vi "Periodic Tasks.vi"(8 "error in":errorcluster) -> ()   [LabVIEW 2013]
doc: "This VI runs in parallel to other tasks. It can contain as many user-defined periodic loops as you need. These can carry out PID or other sorts of timed response."
uses:
  <vilib>/Rock Robotics/WPI/DriverStation/WPI_DriverStationRobotMode2.ctl
  <vilib>/Rock Robotics/SystemInterfaces/Utilities/FPGA_UtilitiesLED Source.ctl
  <vilib>/Rock Robotics/SystemInterfaces/Utilities/FPGA_UtilitiesLED State.ctl
  <vilib>/Rock Robotics/WPI/Solenoid/WPI_SolenoidValue.ctl
  <vilib>/Rock Robotics/WPI/Relay/WPI_RelayValue.ctl
  <vilib>/Rock Robotics/WPI/Compressor/WPI_CompressorGetSetRefNum.vi
  Robot Global Data.vi
  <vilib>/Rock Robotics/WPI/Joystick/WPI_JoystickGetSetRefNum.vi
  <vilib>/Rock Robotics/WPI/Solenoid/WPI_SolenoidSetEnum.vi
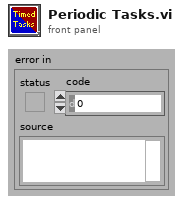
[diagram p1: front panel]
types:
  T1 = typedef "FPGA_UtilitiesLED State.ctl" = enum16{"Off", "On", "Toggle"}
  T2 = typedef "FPGA_UtilitiesLED Source.ctl" = enum16{"User LED", "FPGA LED"}
  T3 = typedef "WPI_AnalogChannelDevRef.ctl" = cluster{"DevStatus":errorcluster, "Analog Module":T4, "Analog Channel":T5}
  T4 = typedef "FPGA_TypedefAnalogModule.ctl" = enum16{"Analog Module 1", "Analog Module 2"}
  T5 = typedef "FPGA_AIChannel.ctl" = enum8{"AI 1", "AI 2", "AI 3", "AI 4", "AI 5", "AI 6", "AI 7", "AI 8", "Invalid"}
  T6 = typedef "WPI_RelayDevRef.ctl" = cluster{"DevStatus":errorcluster, "Relay Channel":T7, "Digital Module":T8, "Relay Direction":T9}
  T7 = typedef "FPGA_DIORelayChannel.ctl" = enum8{"Relay 1", "Relay 2", "Relay 3", "Relay 4", "Relay 5", "Relay 6", "Relay 7", "Relay 8", "Invalid"}
  T8 = typedef "FPGA_TypedefDigitalModule.ctl" = enum16{"Digital Module 1", "Digital Module 2"}
  T9 = typedef "WPI_RelayDirection.ctl" = enum16{"Both directions", "Forward only", "Reverse only"}
  T10 = typedef "WPI_DigitalInputDevRef.ctl" = cluster{"DevStatus":errorcluster, "DIO Channel":T11, "Digital Module":T8}
  T11 = typedef "FPGA_DIOChannel.ctl" = enum8{"DIO 1", "DIO 2", "DIO 3", "DIO 4", "DIO 5", "DIO 6", "DIO 7", "DIO 8", "DIO 9", "DIO 10", "DIO 11", "DIO 12", "DIO 13", "DIO 14", "Invalid"}
  T12 = typedef "WPI_SolenoidDevRef.ctl" = cluster{"DevStatus":errorcluster, "Solenoid Module":T13, "Forward Solenoid Channel":T14, "Reverse Solenoid Channel":T14}
  T13 = typedef "FPGA_TypedefSolenoidModule.ctl" = enum16{"Solenoid Module 1", "Solenoid Module 2"}
  T14 = typedef "WPI_SolenoidChannel.ctl" = enum8{"Solenoid 1", "Solenoid 2", "Solenoid 3", "Solenoid 4", "Solenoid 5", "Solenoid 6", "Solenoid 7", "Solenoid 8", "Invalid"}
  T15 = typedef "WPI_JoystickDevRef.ctl" = cluster{"Device":T16}
  T16 = typedef "WPI_JoystickDeviceEnum.ctl" = enum16{"USB 1", "USB 2", "USB 3", "USB 4", "Kinect 1", "Kinect 2"}
  T17 = typedef "WPI_MotorControlDeviceRef.ctl" = cluster{"DeviceStatus":errorcluster, "Type":enum16{"PWM", "CAN"}, "PWM":cluster{"Digital Module":T8, "PWM Channel":T18, "DeadBand":T19}, "CAN":cluster{"Device Number":u8, "Control Mode":T20, "Semaphore":T21, "Max Vout":dbl}, "Invert":bool, "TransformRef":T22, "InvTransformRef":T22}
  T18 = typedef "FPGA_DIOPWMChannel.ctl" = enum8{"PWM 1", "PWM 2", "PWM 3", "PWM 4", "PWM 5", "PWM 6", "PWM 7", "PWM 8", "PWM 9", "PWM 10", "Invalid"}
  T19 = typedef "WPI_PWMDeadband.ctl" = cluster{"Name":string, "maxPositivePwm":i32, "minPositivePwm":i32, "centerPwm":i32, "maxNegativePwm":i32, "minNegativePwm":i32, "angularRange":u16}
  T20 = typedef "WPI_CANJaguar_ControlMode.ctl" = enum8{"Percent VBus", "Current", "Speed", "Position", "Voltage"}
  T21 = typedef "Semaphore RefNum" = refnum<k1>
  T22 = typedef "WPI_PWMTransform_ConPane.ctl" = refnum<vi>
  T23 = typedef "WPI_CompressorDevRef.ctl" = cluster{"DevStatus":errorcluster, "DigitalInputDevRef":T10, "RelayDevRef":T6}
  T24 = cluster{"JoystickDevRef":T15, "JoystickDevRef":T15, "SolenoidDevRef":T12, "SolenoidDevRef":T12, "RelayDevRef":T6, "RelayDevRef":T6, "RelayDevRef":T6, "MotorControlDevRef":T17, "MotorControlDevRef":T17, "DigitalInputDevRef":T10, "DigitalInputDevRef":T10, "AIDeviceRef":T3, "CompressorDevRef":T23}
  T25 = typedef "WPI_DriverStationRobotMode2.ctl" = enum16{"Autonomous Disabled", "Autonomous Enabled", "Teleop Disabled", "Teleop Enabled", "Timeout", "Finish", "Test Disabled", "Test Enabled"}
  T26 = typedef "WPI_RelayValue.ctl" = enum16{"Off", "On", "Forward", "Reverse"}
  T27 = typedef "WPI_SolenoidValue.ctl" = enum16{"Off", "On", "Forward", "Reverse"}
  T28 = typedef "WPI_JoystickButtonState.ctl" = cluster{"Button 1":bool, "Button 2":bool, "Button 3":bool, "Button 4":bool, "Button 5":bool, "Button 6":bool, "Button 7":bool, "Button 8":bool, "Button 9":bool, "Button 10":bool, "Button 11":bool, "Button 12":bool}
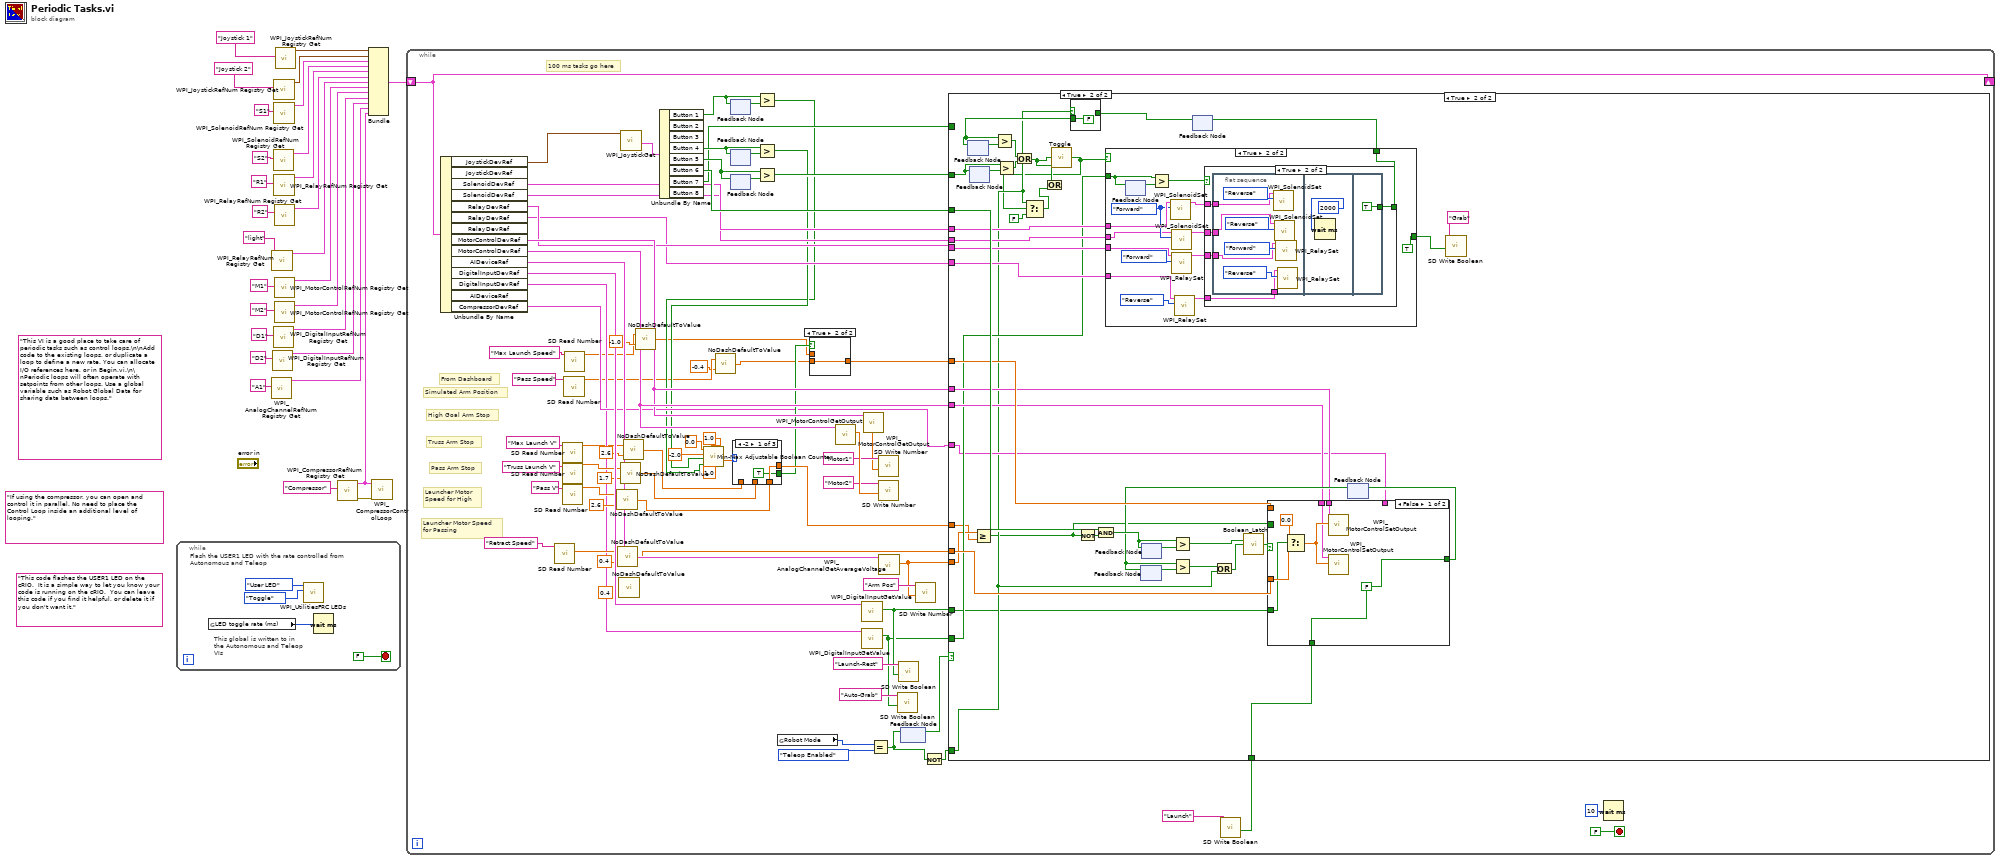
[diagram p0: block diagram]
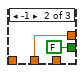
[diagram p3: hidden frame]
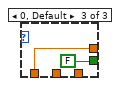
[diagram p4: hidden frame]
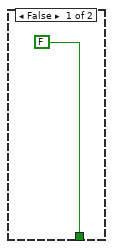
[diagram p5: hidden frame]
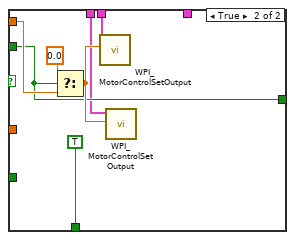
[diagram p7: hidden frame]
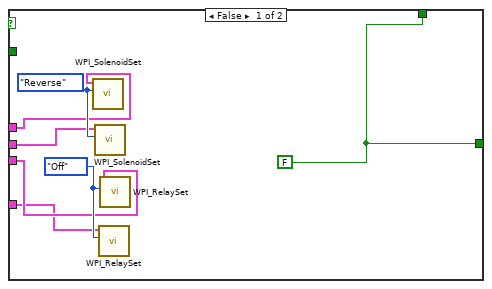
[diagram p8: hidden frame]
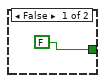
[diagram p9: hidden frame]
diagram:
  (unwired) "If using the compressor, you can open and control it in parallel. No need to place the Control Loop inside an additional level of looping."
  (unwired) "This code flashes the USER1 LED on the cRIO.  It is a simple way to let you know your code is running on the cRIO.  You can leave this code if you find it helpful, or delete it if you don't want it."
  (unwired) "This VI is a good place to take care of periodic tasks such as control loops.\n\nAdd code to the existing loops, or duplicate a loop to define a new rate. You can allocate I/O references here, or in Begin.vi.\n\nPeriodic loops will often operate with setpoints from other loops. Use a global variable such as Robot Global Data for sharing data between loops."
  n1 = while {
    stop <- FALSE stop-if-true
    # "This global is written to in the Autonomous and Teleop VIs"
    # "Flash the USER1 LED with the rate controlled from Autonomous and Teleop"
    n2 = global read "Robot Global Data.vi" "LED toggle rate (ms)"() -> (w29:u32)
    n3 = call <vilib>:"WPI_UtilitiesFRC LEDs.vi"("State"=FPGA_UtilitiesLED_State."Toggle", "LED Type"=FPGA_UtilitiesLED_Source."User LED") -> ()  [unwired: 1 in, 9 out]
    n4 = Wait (ms)(milliseconds to wait=w29) -> ()  [unwired: 1 out]
  }
  n5 = call <vilib>:"WPI_AnalogChannelRefNum Registry Get.vi"("refnum name"="A1") -> ("AIDeviceRef"=w2:T3)  [unwired: 9 in, 1 out]
  n6 = call <vilib>:"WPI_RelayRefNum Registry Get.vi"("refnum name"="light") -> ("RelayDevRef"=w10:T6)  [unwired: 9 in, 1 out]
  n7 = call <vilib>:"WPI_DigitalInputRefNum Registry Get.vi"("refnum name"="D2") -> ("DigitalInputDevRef"=w3:T10)  [unwired: 9 in, 1 out]
  n8 = call <vilib>:"WPI_SolenoidRefNum Registry Get.vi"("refnum name"="S2") -> ("SolenoidDevRef"=w13:T12)  [unwired: 9 in, 1 out]
  n9 = call <vilib>:"WPI_DigitalInputRefNum Registry Get.vi"("refnum name"="D1") -> ("DigitalInputDevRef"=w7:T10)  [unwired: 9 in, 1 out]
  n10 = call <vilib>:"WPI_JoystickRefNum Registry Get.vi"("refnum name"="Joystick 2") -> ("JoystickDevRef"=w5:T15)  [unwired: 1 in, 9 out]
  n11 = call <vilib>:"WPI_SolenoidRefNum Registry Get.vi"("refnum name"="S1") -> ("SolenoidDevRef"=w4:T12)  [unwired: 9 in, 1 out]
  n12 = call <vilib>:"WPI_RelayRefNum Registry Get.vi"("refnum name"="R1") -> ("RelayDevRef"=w12:T6)  [unwired: 9 in, 1 out]
  n13 = call <vilib>:"WPI_RelayRefNum Registry Get.vi"("refnum name"="R2") -> ("RelayDevRef"=w11:T6)  [unwired: 9 in, 1 out]
  n14 = call <vilib>:"WPI_MotorControlRefNum Registry Get.vi"("refnum name"="M1") -> ("MotorControlDevRef"=w9:T17)  [unwired: 9 in, 1 out]
  n15 = call <vilib>:"WPI_MotorControlRefNum Registry Get.vi"("refnum name"="M2") -> ("MotorControlDevRef"=w8:T17)  [unwired: 9 in, 1 out]
  n16 = call <vilib>:"WPI_JoystickRefNum Registry Get.vi"("refnum name"="Joystick 1") -> ("JoystickDevRef"=w6:T15)  [unwired: 1 in, 9 out]
  n17 = call <vilib>:"WPI_CompressorRefNum Registry Get.vi"("refnum name"="Compressor") -> ("error out"=w15:errorcluster, "CompressorDevRef"=w1:T23)  [unwired: 9 in]
  n18 = Bundle("JoystickDevRef"=w6, "JoystickDevRef"=w5, "SolenoidDevRef"=w4, "SolenoidDevRef"=w13, "RelayDevRef"=w12, "RelayDevRef"=w11, "RelayDevRef"=w10, "MotorControlDevRef"=w9, "MotorControlDevRef"=w8, "DigitalInputDevRef"=w7, "DigitalInputDevRef"=w3, "AIDeviceRef"=w2, "CompressorDevRef"=w1) -> (w27:T24)  [unwired: 1 out]
  n19 = call <vilib>:"WPI_CompressorControlLoop.vi"("error in (no error)"=w15, "CompressorDevRef"=w1) -> ()  [unwired: 10 in]
  n20 = while {
    shift-right: [w106] -> _
    shift-left: w27 -> [w106]
    stop <- FALSE stop-if-true
    (unwired) 0.4
    # "Simulated Arm Position"
    # "Launcher Motor Speed\nfor Passing"
    # "Launcher Motor\nSpeed for High"
    # "Pass Arm Stop"
    # "Truss Arm Stop"
    # "High Goal Arm Stop"
    # "From Dashboard"
    # "100 ms tasks go here"
    n21 = Unbundle By Name(w106) -> ("JoystickDevRef"=w105:T15, "SolenoidDevRef"=w70:T12, "SolenoidDevRef"=w68:T12, "RelayDevRef"=w65:T6, "RelayDevRef"=w64:T6, "MotorControlDevRef"=w87:T17, "MotorControlDevRef"=w88:T17, "AIDeviceRef"=w91:T3, "DigitalInputDevRef"=w92:T10, "DigitalInputDevRef"=w43:T10, "CompressorDevRef"=w60:T23)  [unwired: 3 out]
    n22 = call <vilib>:"SD Read Number.vi"("Name"="Retract Speed") -> ("Numeric"=w50:dbl)  [unwired: 8 in, 2 out]
    n23 = call <vilib>:"SD Read Number.vi"("Name"="Max Launch V") -> ("Numeric"=w41:dbl)  [unwired: 8 in, 2 out]
    n24 = call <vilib>:"SD Read Number.vi"("Name"="Truss Launch V") -> ("Numeric"=w45:dbl)  [unwired: 8 in, 2 out]
    n25 = call <vilib>:"SD Read Number.vi"("Name"="Pass V") -> ("Numeric"=w47:dbl)  [unwired: 8 in, 2 out]
    n26 = call <vilib>:"SD Read Number.vi"("Name"="Pass Speed") -> ("Numeric"=w35:dbl)  [unwired: 8 in, 2 out]
    n27 = call <vilib>:"SD Read Number.vi"("Name"="Max Launch Speed") -> ("Numeric"=w37:dbl)  [unwired: 8 in, 2 out]
    n28 = call "NoDashDefaultToValue.vi"("Numeric 2"=2.6, "Numeric"=w47) -> ("Numeric 3"=w46:dbl)
    n29 = call "NoDashDefaultToValue.vi"("Numeric 2"=0.4, "Numeric"=w50) -> ("Numeric 3"=w49:dbl)
    n30 = call "NoDashDefaultToValue.vi"() -> ()  [unwired: 2 in, 1 out]
    n31 = call "NoDashDefaultToValue.vi"("Numeric 2"=1.7, "Numeric"=w45) -> ("Numeric 3"=w44:dbl)
    n32 = call <vilib>:"WPI_JoystickGet.vi"("JoystickDevRef"=w105) -> ("Buttons"=w104:T28)  [unwired: 4 in, 2 out]
    n33 = call "NoDashDefaultToValue.vi"("Numeric 2"=2.6, "Numeric"=w41) -> ("Numeric 3"=w40:dbl)
    n34 = call "NoDashDefaultToValue.vi"("Numeric 2"=-1.0, "Numeric"=w37) -> ("Numeric 3"=w36:dbl)
    n35 = Unbundle By Name(w104) -> ("Button 1"=w102:bool, "Button 4"=w100:bool, "Button 5"=w98:bool, "Button 6"=w82:bool, "Button 7"=w69:bool)  [unwired: 3 out]
    n36 = call "NoDashDefaultToValue.vi"("Numeric 2"=-0.4, "Numeric"=w35) -> ("Numeric 3"=w33:dbl)
    n37 = feedback #1() -> (w103:bool)  [unwired: 1 in]
    n38 = feedback-in #1(w102) -> ()
    n39 = feedback #2() -> (w101:bool)  [unwired: 1 in]
    n40 = feedback-in #2(w100) -> ()
    n41 = feedback #3() -> (w99:bool)  [unwired: 1 in]
    n42 = feedback-in #3(w98) -> ()
    n43 = Greater?(x=w102, y=w103) -> (0:w58:bool)
    n44 = Greater?(x=w100, y=w101) -> (0:w59:bool)
    n45 = call "Min-Max Adjustable Boolean Counter.vi"("Dec Amount"=1.0, "Inc Amount"=1.0, "Decrease"=w58, "Increase"=w59, "Minimum"=-2.0, "Maximum"=0.0) -> ("Counter"=w53:dbl)  [unwired: 5 in]
    n46 = case shown="-2" w53 {
      tunnel: w46 -> [w111 _ _]
      tunnel: w44 -> [_ w113 _]
      tunnel: w40 -> [_ _ w115]
      tunnel: [w111 w113 w115] -> w76
      tunnel: [TRUE FALSE FALSE] -> w66
      frame -2 {
      }
      frame -1 {
      }
      frame 0, Default {
      }
    }
    n47 = Greater?(x=w98, y=w99) -> (0:w97:bool)
    n48 = global read "Robot Global Data.vi" "Robot Mode"() -> (w72:T25)
    n49 = case shown="True" w66 {
      tunnel: w33 -> [_ w109]
      tunnel: [w108 w109] -> w75
      tunnel: w36 -> [w108 _]
      frame False {
      }
      frame True {
      }
    }
    n50 = call <vilib>:"WPI_MotorControlGetOutput.vi"("MotorControlDevRef"=w88) -> ("Output"=w86:dbl)  [unwired: 8 in, 2 out]
    n51 = call <vilib>:"WPI_DigitalInputGetValue.vi"("DigitalInputDevRef"=w92) -> ("Value"=w94:bool)  [unwired: 8 in, 2 out]
    n52 = call <vilib>:"WPI_DigitalInputGetValue.vi"("DigitalInputDevRef"=w43) -> ("Value"=w93:bool)  [unwired: 8 in, 2 out]
    n53 = call <vilib>:"WPI_MotorControlGetOutput.vi"("MotorControlDevRef"=w87) -> ("Output"=w84:dbl)  [unwired: 8 in, 2 out]
    n54 = Equal?(x=w72, y=WPI_DriverStationRobotMode2."Teleop Enabled") -> (x = y?=w61:bool)
    n55 = call <vilib>:"SD Write Number.vi"("Numeric"=w84, "Name"="Motor1") -> ()  [unwired: 8 in, 2 out]
    n56 = call <vilib>:"SD Write Number.vi"("Numeric"=w86, "Name"="Motor2") -> ()  [unwired: 8 in, 2 out]
    n57 = call <vilib>:"WPI_AnalogChannelGetAverageVoltage.vi"("AIDeviceRef"=w91) -> ("Voltage"=w89:dbl)  [unwired: 8 in, 2 out]
    n58 = call <vilib>:"SD Write Boolean.vi"("Boolean"=w93, "Name"="Auto-Grab") -> ()  [unwired: 8 in, 2 out]
    n59 = call <vilib>:"SD Write Boolean.vi"("Boolean"=w94, "Name"="Launch-Rest") -> ()  [unwired: 8 in, 2 out]
    n60 = feedback-in #4(w61) -> ()
    n61 = feedback #4() -> (w63:bool)  [unwired: 1 in]
    n62 = call <vilib>:"SD Write Number.vi"("Numeric"=w89, "Name"="Arm Pos") -> ()  [unwired: 8 in, 2 out]
    n63 = Not(x=w61) -> (.not. x?=w62:bool)
    n64 = case shown="True" w63 {
      tunnel: w97 -> [_ w156]
      tunnel: w94 -> [_ w122]
      tunnel: w93 -> [_ w129]
      tunnel: w89 -> [_ w127]
      tunnel: w88 -> [_ w140]
      tunnel: w87 -> [_ w141]
      tunnel: w82 -> [_ w152]
      tunnel: w76 -> [_ w126]
      tunnel: w75 -> [_ w151]
      tunnel: [FALSE w147] -> w73
      tunnel: w70 -> [_ w139]
      tunnel: w69 -> [_ _]
      tunnel: w68 -> [_ w137]
      tunnel: w49 -> [_ w138]
      tunnel: w65 -> [_ w136]
      tunnel: w64 -> [_ w135]
      tunnel: w62 -> [_ w125]
      tunnel: w60 -> [_ w128]
      frame False {
      }
      frame True {
        n65 = feedback #5() -> (w144:bool)  [unwired: 1 in]
        n66 = feedback #6() -> (w157:bool)  [unwired: 1 in]
        n67 = feedback-in #6(w156) -> ()
        n68 = Greater Or Equal?(x=w127, y=w126) -> (x >= y?=w123:bool)
        n69 = Greater?(x=w156, y=w157) -> (0:w133:bool)
        n70 = Not(x=w123) -> (.not. x?=w153:bool)
        n71 = And(x=w152, y=w153) -> (x .and. y?=w154:bool)
        n72 = feedback #7() -> (w149:bool)  [unwired: 1 in]
        n73 = feedback #8() -> (w155:bool)  [unwired: 1 in]
        n74 = feedback-in #8(w154) -> ()
        n75 = Greater?(x=w154, y=w155) -> (0:w121:bool)
        n76 = feedback #9() -> (w131:bool)  [unwired: 1 in]
        n77 = case shown="True" w125 {
          tunnel: w131 -> [w158 _]
          tunnel: [w158 FALSE] -> w130
          frame False {
          }
          frame True {
          }
        }
        n78 = feedback-in #5(w130) -> ()
        n79 = Greater?(x=w130, y=w144) -> (0:w143:bool)
        n80 = Or(x=w143, y=w133) -> (x .or. y?=w118:bool)
        n81 = call "Toggle.vi"("Input"=w118) -> ("Output"=w117:bool)
        n82 = Select(t=w125, s=w117, f=FALSE) -> (s? t:f=w132:bool)
        n83 = Or(x=w118, y=w132) -> ()  [unwired: 1 out]
        n84 = case shown="True" w117 {
          tunnel: [w179 TRUE] -> w145
          tunnel: [w179 w189] -> w142
          tunnel: w139 -> [w177 w187]
          tunnel: w137 -> [w176 w185]
          tunnel: w136 -> [w175 w184]
          tunnel: w135 -> [w174 w183]
          tunnel: w129 -> [_ w182]
          frame False {
            w180 = WPI_RelayValue."Off" ("RelayValue")
            w179 = FALSE
            w178 = WPI_SolenoidValue."Reverse" ("Value")
            n85 = call-poly <vilib>:"WPI_SolenoidSet.vi"("Value"=w178, "SolenoidDevRef"=w177) -> ()  [unwired: 8 in, 2 out]
            n86 = call-poly <vilib>:"WPI_SolenoidSet.vi"("Value"=w178, "SolenoidDevRef"=w176) -> ()  [unwired: 8 in, 2 out]
            n87 = call <vilib>:"WPI_RelaySet.vi"("RelayValue"=w180, "RelayDevRef"=w174) -> ()  [unwired: 8 in, 2 out]
            n88 = call <vilib>:"WPI_RelaySet.vi"("RelayValue"=w180, "RelayDevRef"=w175) -> ()  [unwired: 8 in, 2 out]
          }
          frame True {
            w186 = WPI_SolenoidValue."Forward" ("Value")
            n89 = feedback #10() -> (w181:bool)  [unwired: 1 in]
            n90 = feedback-in #10(w182) -> ()
            n91 = Greater?(x=w182, y=w181) -> (0:w188:bool)
            n92 = call-poly <vilib>:"WPI_SolenoidSet.vi"("Value"=w186, "SolenoidDevRef"=w187) -> ("SolenoidDevRef"=w193:T12)  [unwired: 8 in, 1 out]
            n93 = call-poly <vilib>:"WPI_SolenoidSet.vi"("Value"=w186, "SolenoidDevRef"=w185) -> ("SolenoidDevRef"=w192:T12)  [unwired: 8 in, 1 out]
            n94 = call <vilib>:"WPI_RelaySet.vi"("RelayValue"=WPI_RelayValue."Forward", "RelayDevRef"=w184) -> ("RelayDevRef"=w191:T6)  [unwired: 8 in, 1 out]
            n95 = call <vilib>:"WPI_RelaySet.vi"("RelayValue"=WPI_RelayValue."Reverse", "RelayDevRef"=w183) -> ("RelayDevRef"=w190:T6)  [unwired: 8 in, 1 out]
            n96 = case shown="True" w188 {
              tunnel: w193 -> [_ w202]
              tunnel: w192 -> [_ w201]
              tunnel: w191 -> [_ w200]
              tunnel: w190 -> [_ w199]
              tunnel: [FALSE w198] -> w189
              frame False {
              }
              frame True {
                n97 = flat-sequence {
                  tunnel: w202 -> [w206]
                  tunnel: w201 -> [w205]
                  tunnel: w200 -> [w204]
                  tunnel: w199 -> [w203]
                  tunnel: [TRUE] -> w198
                  frame #0 {
                    n98 = call-poly <vilib>:"WPI_SolenoidSet.vi"("Value"=WPI_SolenoidValue."Reverse", "SolenoidDevRef"=w206) -> ()  [unwired: 8 in, 2 out]
                    n99 = call-poly <vilib>:"WPI_SolenoidSet.vi"("Value"=WPI_SolenoidValue."Reverse", "SolenoidDevRef"=w205) -> ()  [unwired: 8 in, 2 out]
                    n100 = call <vilib>:"WPI_RelaySet.vi"("RelayValue"=WPI_RelayValue."Forward", "RelayDevRef"=w204) -> ()  [unwired: 8 in, 2 out]
                    n101 = call <vilib>:"WPI_RelaySet.vi"("RelayValue"=WPI_RelayValue."Reverse", "RelayDevRef"=w203) -> ()  [unwired: 8 in, 2 out]
                  }
                  frame #1 {
                    n102 = Wait (ms)(milliseconds to wait=2000) -> ()  [unwired: 1 out]
                  }
                  frame #2 {
                  }
                }
              }
            }
          }
        }
        n103 = feedback-in #9(w142) -> ()
        n104 = feedback #11() -> (w148:bool)  [unwired: 1 in]
        n105 = feedback-in #7(w148) -> ()
        n106 = Greater?(x=w148, y=w149) -> (0:w124:bool)
        n107 = Or(x=w124, y=w125) -> (x .or. y?=w120:bool)
        n108 = call "Boolean_Latch.vi"("Latch Control"=w121, "Reset"=w120) -> ("Latched?"=w119:bool)  [unwired: 13 in]
        n109 = case shown="False" w119 {
          tunnel: w151 -> [_ w172]
          tunnel: w123 -> [_ w170]
          tunnel: [w164 w170] -> w150
          tunnel: [w164 TRUE] -> w147
          tunnel: w141 -> [w162 w168]
          tunnel: w140 -> [w161 w167]
          tunnel: w138 -> [w163 _]
          tunnel: w128 -> [_ _]
          tunnel: w122 -> [w160 _]
          frame False {
            w164 = FALSE
            n110 = Select(t=0.0, s=w160, f=w163) -> (s? t:f=w165:dbl)
            n111 = call <vilib>:"WPI_MotorControlSetOutput.vi"("Output"=w165, "MotorControlDevRef"=w162) -> ()  [unwired: 7 in, 3 out]
            n112 = call <vilib>:"WPI_MotorControlSetOutput.vi"("Output"=w165, "MotorControlDevRef"=w161) -> ()  [unwired: 7 in, 3 out]
          }
          frame True {
            n113 = Select(t=0.0, s=w170, f=w172) -> (s? t:f=w173:dbl)
            n114 = call <vilib>:"WPI_MotorControlSetOutput.vi"("Output"=w173, "MotorControlDevRef"=w168) -> ()  [unwired: 7 in, 3 out]
            n115 = call <vilib>:"WPI_MotorControlSetOutput.vi"("Output"=w173, "MotorControlDevRef"=w167) -> ()  [unwired: 7 in, 3 out]
          }
        }
        n116 = feedback-in #11(w150) -> ()
        n117 = call <vilib>:"SD Write Boolean.vi"("Boolean"=w145, "Name"="Grab") -> ()  [unwired: 8 in, 2 out]
      }
    }
    n118 = call <vilib>:"SD Write Boolean.vi"("Boolean"=w73, "Name"="Launch") -> ()  [unwired: 8 in, 2 out]
    n119 = Wait (ms)(milliseconds to wait=u32 10) -> ()  [unwired: 1 out]
  }
